vi "Set Abort.vi"(8 "error in (no error)":errorcluster {"code" format="Error %.0f"}, 10 "Abort?":bool, 11 "Progress Bar UI In":refnum<class "Progress Bar UI.lvclass">) -> (0 "error out":errorcluster {"code" format="Error %.0f"}, 3 "Progress Bar UI Out":refnum<class "Progress Bar UI.lvclass">)   [LabVIEW 2023, in "Progress Bar UI.lvclass"]
uses:
  Progress Bar UI.lvclass
  Progress Bar UI.lvclass/Progress Bar UI.ctl
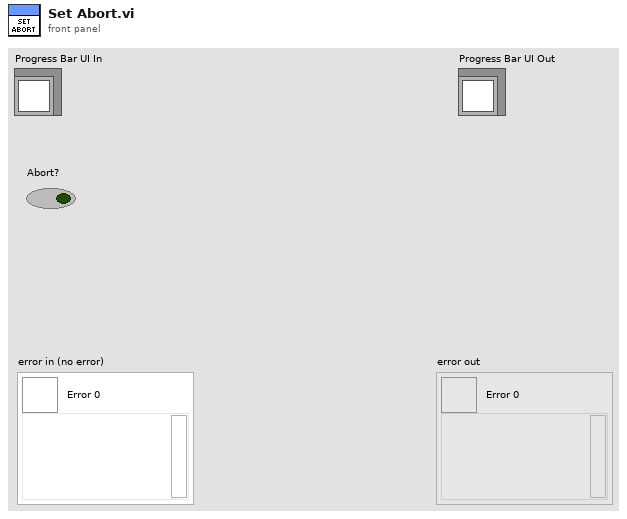
[diagram p1: front panel]
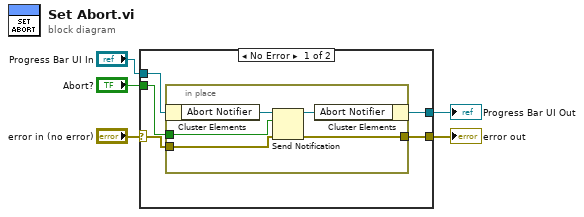
[diagram p0: block diagram]
diagram:
  n1 = case shown="No Error" "error in (no error)" {
    selector: "error in (no error)" -> [w8 w17]
    tunnel: [w7 w17] -> w4
    tunnel: [w10 w16] -> w2
    tunnel: "Progress Bar UI In" -> [w9 w16]
    tunnel: "Abort?" -> [w6 _]
    frame No Error {
      n2 = in-place {
        in-place-border: w6 -> [w13]
        in-place-border: w8 -> [w12]
        in-place-border: [w11] -> w7
        n3 = in-place-cluster #1(w9) -> ("Abort Notifier"=w15:refnum<notifier>)
        n4 = Send Notification(notification=w13, notifier=w15, error in (no error)=w12) -> (notifier out=w14:refnum<notifier>, error out=w11:errorcluster)
        n5 = in-place-cluster #1("Abort Notifier"=w14) -> (w10:refnum<class "Progress Bar UI.lvclass">)
      }
    }
    frame Error {
    }
  }
  "error out" <- w4
  "Progress Bar UI Out" <- w2
